vi "File Page.vi"(8 "error in (no error)":errorcluster, 11 "Node Ptr":T1 format="%.0x") -> (0 "error out":errorcluster)   [LabVIEW 2020, in "Telemetry System Explorer.lvlib"]
uses:
  Telemetry System Explorer.lvlib
  <vilib>/NI VeriStand/Custom Device API/Custom Device API.lvlib
  Shared/Constants.vi
  Shared/Telemetry Shared.lvlib
  <vilib>/NI VeriStand/Custom Device API/Set Item Property (Boolean).vi
  <vilib>/NI VeriStand/Custom Device API/Custom Device Item Ref.ctl
panel:
  out "Log File Path for RT Targets":path
  out "Log File Path for Windows Targets":path
  in  "Overwrite File If Exists?":bool
  in  "SHDocVw.IWebBrowser":refnum<k7>(container)
  in  "Specific Header":cluster{"Section Name":string}={"Section Name"="Log File Specification"}
  in  "General Header":cluster{"Section Name":string}={"Section Name"="Log Section Settings"}
  in  "Description":string
  in  "Name":string
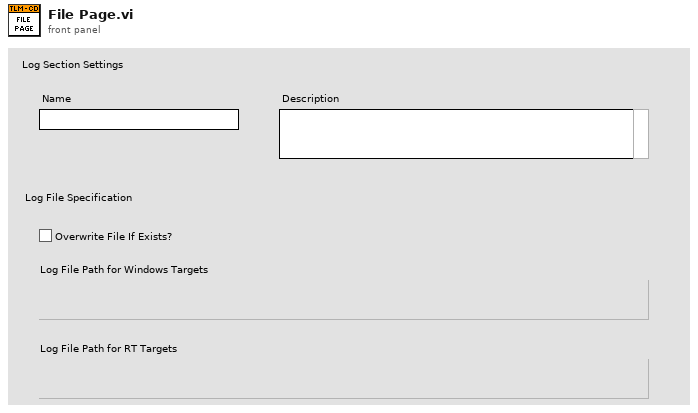
[diagram p1: front panel]
types:
  T1 = typedef "Custom Device API.lvlib/Custom Device Item Ref.ctl" = u64
  T2 = typedef "Custom Device API.lvlib/Custom Device Item Info.ctl" = cluster{"Name":string, "Is Channel":bool, "GUID":string, "Is Waveform":bool}
  T3 = typedef "Custom Device API.lvlib/Custom Device Commands.ctl" = enum16{"Default", "Item renamed", "Shutdown", "Dynamic button pressed"}
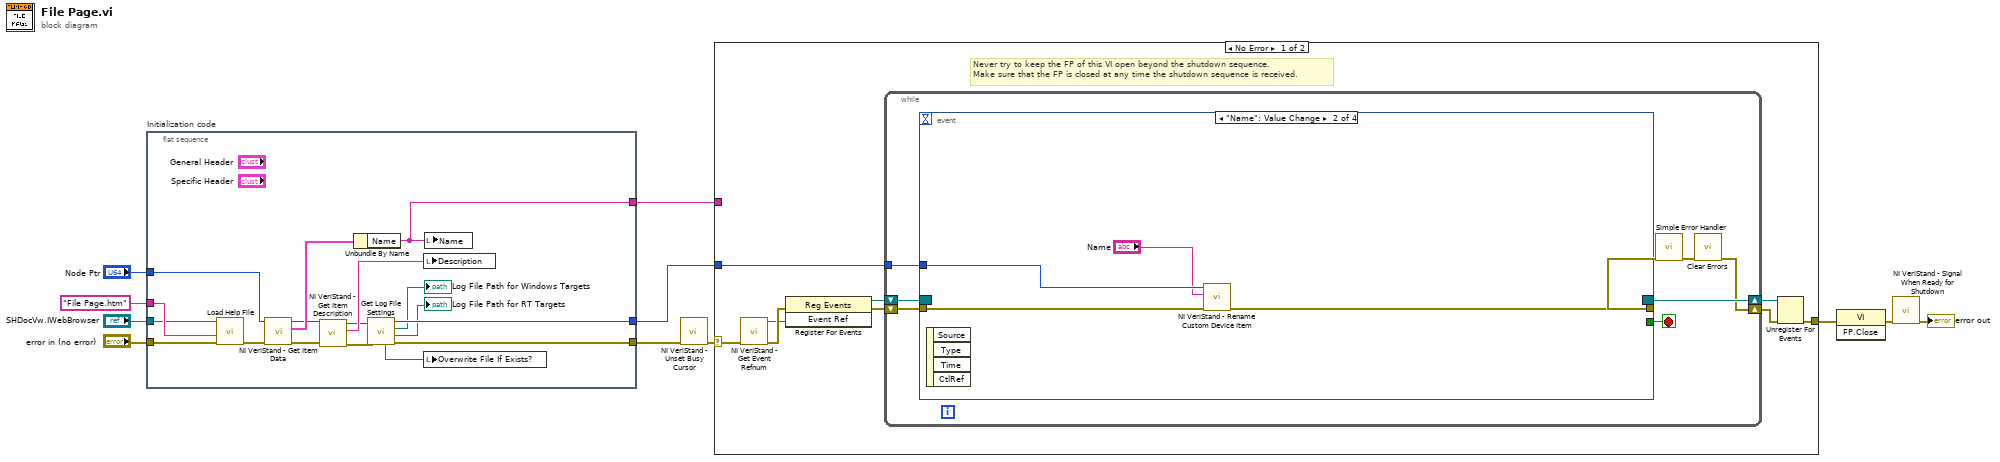
[diagram p0: block diagram]
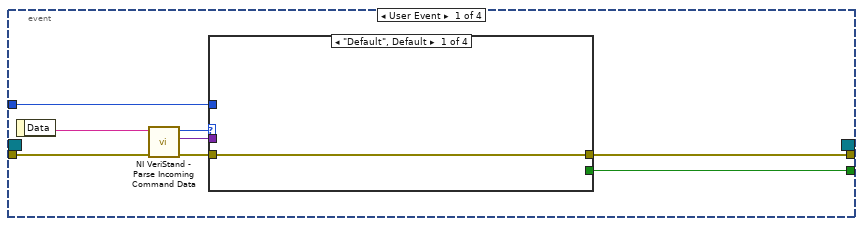
[diagram p2: hidden frame]
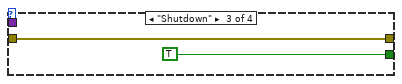
[diagram p4: hidden frame]
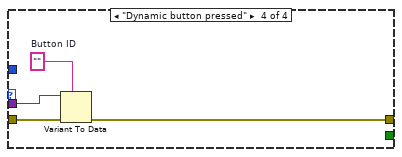
[diagram p5: hidden frame]
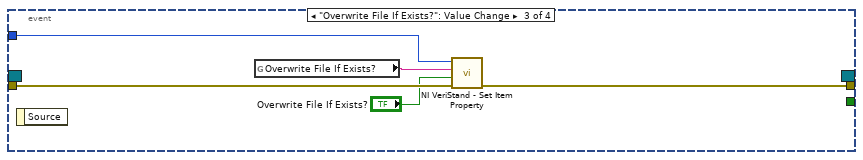
[diagram p6: hidden frame]
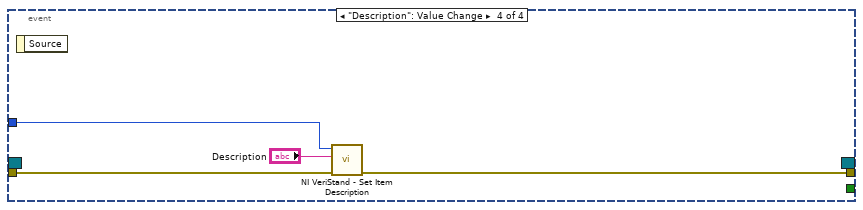
[diagram p7: hidden frame]
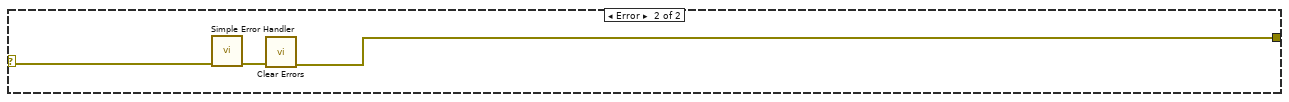
[diagram p8: hidden frame]
diagram:
  n1 = flat-sequence "Initialization code" {
    tunnel: "error in (no error)" -> [w27]
    tunnel: "Node Ptr" -> [w18]
    tunnel: [w23] -> w7
    tunnel: [w24] -> w4
    tunnel: "SHDocVw.IWebBrowser" -> [w25]
    tunnel: "File Page.htm" ("CD_CHM_Section") -> [w26]
    tunnel: [w15] -> w1
    frame #0 {
      n2 = call "Load Help File.vi"("error in (no error)"=w27, "HTML File to Load"=w26, "Browser"=w25) -> ("error out"=w21:errorcluster)  [unwired: 8 in]
      n3 = call <vilib>:"NI VeriStand - Get Item Data.vi"("error in (no error)"=w21, "Item Ref in"=w18) -> ("error out"=w20:errorcluster, "Item Info"=w22:T2, "Item Ref out"=w17:T1)  [unwired: 7 out]
      n4 = call <vilib>:"NI VeriStand - Get Item Description.vi"("error in (no error)"=w20, "Item Ref in"=w17) -> ("error out"=w19:errorcluster, "Description"=w28:string, "Item Ref out"=w16:T1)  [unwired: 7 out]
      n5 = Unbundle By Name(w22) -> ("Name"=w15:string)
      n6 = call "Get Log File Settings.vi"("error in (no error)"=w19, "File Ref in"=w16) -> ("error out"=w23:errorcluster, "File Path - RT Targets"=→"Log File Path for RT Targets":path, "File Path - Windows"=→"Log File Path for Windows Targets":path, "File Ref out"=w24:T1, "Ovewrite File If Exists?"=w14:bool)  [unwired: 5 in]
      n7 = local write "Description"(w28) -> ()
      n8 = local write "Overwrite File If Exists?"(w14) -> ()
      n9 = local write "Name"(w15) -> ()
    }
  }
  n10 = call <vilib>:"NI VeriStand - Unset Busy Cursor.vi"("error in (no error)"=w7) -> ("error out"=w6:errorcluster)  [unwired: 10 out]
  n11 = case shown="No Error" w6 {
    selector: w6 -> [w29 w77]
    tunnel: [w34 w75] -> w11
    tunnel: w4 -> [w30 _]
    tunnel: w1 -> [_ _]
    frame No Error {
      # "Never try to keep the FP of this VI open beyond the shutdown sequence.\nMake sure that the FP is closed at any time the shutdown sequence is received."
      n12 = call <vilib>:"NI VeriStand - Get Event Refnum.vi"("error in (no error)"=w29) -> ("error out"=w37:errorcluster, "Event Ref"=w33:refnum<user-event>)  [unwired: 9 out]
      n13 = register-events(error in=w37, w33) -> (reference out=w31:refnum<event-registration>, error out=w32:errorcluster)  [unwired: 1 in]
      n14 = while {
        tunnel: w30 -> [w41]
        shift-right: [w38] -> w35
        shift-left: w32 -> [w44]
        shift-right: [w45] -> w36
        shift-left: w31 -> [w43]
        stop <- w42 stop-if-true
        n15 = event shown="[1] \"Name\": Value Change" {
          selector: w43 -> [_ _ _ _]
          dyn-events: [_ _ _ _] -> w45
          timeout: _ -> [_ _ _ _]
          tunnel: w44 -> [w53 w65 w70 w73]
          tunnel: [w49 _ _ _] -> w42
          tunnel: [w48 w62 w69 w72] -> w40
          tunnel: w41 -> [w46 w64 w68 w74]
          event User Event {
            n16 = event-data() -> ("Data"=w52:string)  [unwired: 1 out]
            n17 = call <vilib>:"NI VeriStand - Parse Incoming Command Data.vi"("error in (no error)"=w53, "Incoming data"=w52) -> ("error out"=w51:errorcluster, "Outgoing data"=w47:variant, "Action"=w50:T3)  [unwired: 7 out]
            n18 = case shown="\"Default\", Default" w50 {
              tunnel: w51 -> [w54 w55 w56 w61]
              tunnel: [_ _ TRUE _] -> w49
              tunnel: [w54 w55 w56 w58] -> w48
              tunnel: w46 -> [_ _ _ _]
              tunnel: w47 -> [_ _ _ w60]
              frame "Default", Default {
              }
              frame "Item renamed" {
              }
              frame "Shutdown" {
              }
              frame "Dynamic button pressed" {
                w59 = ""  # Button ID
                n19 = Variant To Data(error in=w61, type=w59, Variant=w60) -> (error out=w58:errorcluster)  [unwired: 1 out]
              }
            }
          }
          event "Name": Value Change {
            n20 = event-data() -> ()  [unwired: 5 out]
            n21 = call <vilib>:"NI VeriStand - Rename Custom Device Item.vi"("error in (no error)"=w65, "New Name"="Name", "Item Ref in"=w64) -> ("error out"=w62:errorcluster)  [unwired: 1 in, 7 out]
          }
          event "Overwrite File If Exists?": Value Change {
            n22 = event-data() -> ()  [unwired: 2 out]
            n23 = global read "Constants.vi" "Overwrite File If Exists?"() -> (w67:string)
            n24 = call-poly <vilib>:"NI VeriStand - Set Item Property.vi"("error in (no error)"=w70, "Value"="Overwrite File If Exists?", "Property Name"=w67, "Item Ref in"=w68) -> ("error out"=w69:errorcluster)  [unwired: 5 in, 2 out]
          }
          event "Description": Value Change {
            n25 = event-data() -> ()  [unwired: 2 out]
            n26 = call <vilib>:"NI VeriStand - Set Item Description.vi"("error in (no error)"=w73, "Description"="Description", "Item Ref in"=w74) -> ("error out"=w72:errorcluster)  [unwired: 8 out]
          }
        }
        n27 = call <vilib>:"Simple Error Handler.vi"("error in (no error)"=w40) -> ("error out"=w39:errorcluster)  [unwired: 1 in, 7 out]
        n28 = call <vilib>:"Clear Errors.vi"("error in (no error)"=w39) -> ("error out"=w38:errorcluster)  [unwired: 1 in, 5 out]
      }
      n29 = Unregister For Events(event registration refnum=w36, error in=w35) -> (error out=w34:errorcluster)
    }
    frame Error {
      n30 = call <vilib>:"Simple Error Handler.vi"("error in (no error)"=w77) -> ("error out"=w76:errorcluster)  [unwired: 1 in, 7 out]
      n31 = call <vilib>:"Clear Errors.vi"("error in (no error)"=w76) -> ("error out"=w75:errorcluster)  [unwired: 1 in, 5 out]
    }
  }
  n32 = invoke class="VI" method="FP.Close"(error in=w11) -> (error out=w10:errorcluster)  [unwired: 2 in, 2 out]
  n33 = call <vilib>:"NI VeriStand - Signal When Ready for Shutdown.vi"("error in (no error)"=w10) -> ("error out"=→"error out":errorcluster)  [unwired: 10 out]
